vi "writeSALCommand.vi"(8 "error in":errorcluster, 10 "Command.lvclass":refnum<class "Command.lvclass">, 11 "SALCommand.lvclass in":refnum<class "SALCommand.lvclass">) -> (0 "error out":errorcluster, 3 "SALCommand.lvclass out":refnum<class "SALCommand.lvclass">)   [LabVIEW 2016, in "SALCommand.lvclass"]
uses:
  SALCommand.lvclass
  ComponentTemplateCore/ComponentModel/ComponentModel/Command/Command.lvclass
  SALCommand.lvclass/SALCommand.ctl
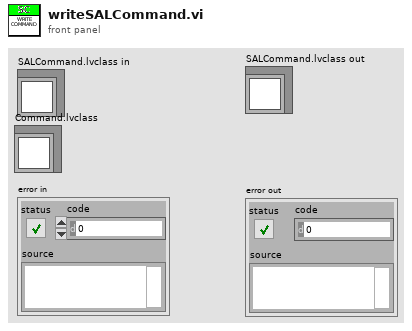
[diagram p1: front panel]
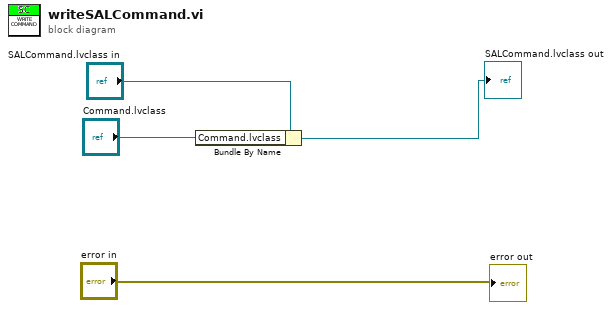
[diagram p0: block diagram]
diagram:
  n1 = Bundle By Name(cluster="SALCommand.lvclass in", "Command.lvclass"="Command.lvclass") -> (→"SALCommand.lvclass out":refnum<class "SALCommand.lvclass">)
  "error out" <- "error in"
